vi "Unflatten Value.vi"(8 "Error In":errorcluster, 10 "Value":string, 11 "Path In":refnum<class "Path.lvclass">) -> (0 "Error Out":errorcluster, 3 "Path Out":refnum<class "Path.lvclass">)   [LabVIEW 2017, in "Tree API.lvlib" / "Path.lvclass"]
uses:
  Path.lvclass
  Tree Manager/Tree.lvclass
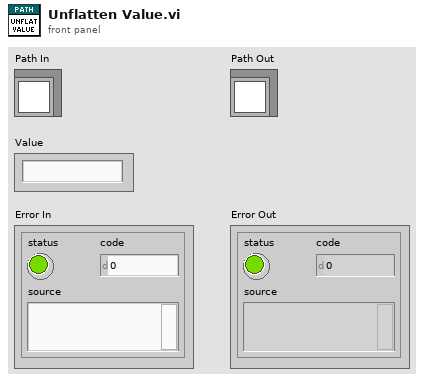
[diagram p1: front panel]
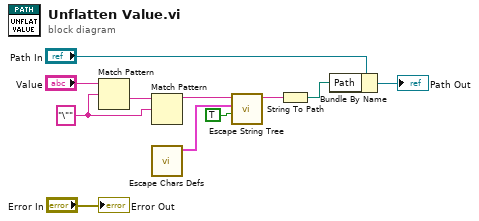
[diagram p0: block diagram]
diagram:
  w5 = "\"" ("regular expression")
  n1 = Match Pattern(string="Value", regular expression=w5) -> (after substring=w6:string)  [unwired: 1 in, 3 out]
  n2 = Match Pattern(string=w6, regular expression=w5) -> (before substring=w3:string)  [unwired: 1 in, 3 out]
  n3 = call "Escape Chars Defs.vi"() -> ("Escapes"=w4:cluster{"String":string, "Escape":string}[])  [unwired: 11 in]
  n4 = call "Escape String Tree.vi"("Reverse? (False)"=TRUE, "Escapes"=w4, "String In"=w3) -> ("String Out"=w1:string)  [unwired: 8 in]
  n5 = String To Path(string=w1) -> (path=w9:path)
  n6 = Bundle By Name(cluster="Path In", "Path"=w9) -> (→"Path Out":refnum<class "Path.lvclass">)
  "Error Out" <- "Error In"
